vi "Select INSTR Dialog.vi"() -> (0 "Cancel":bool, 1 "element":string)   [LabVIEW 2010]
doc: "This VI scans for connected USB test and measurement devices. All found devices are shown in a list, where the user can select one of the connected devices. \nOK initialice selected device\nRESCAN look again for connected devices \nCANCEL abort application"
panel:
  in  "Rescan":bool
  in  "Cancel Button":bool
  in  "OK":bool
  in  "Select":i32(listbox) caption="Select Device from List and Press OK"
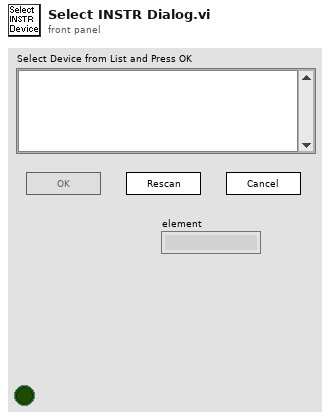
[diagram p1: front panel]
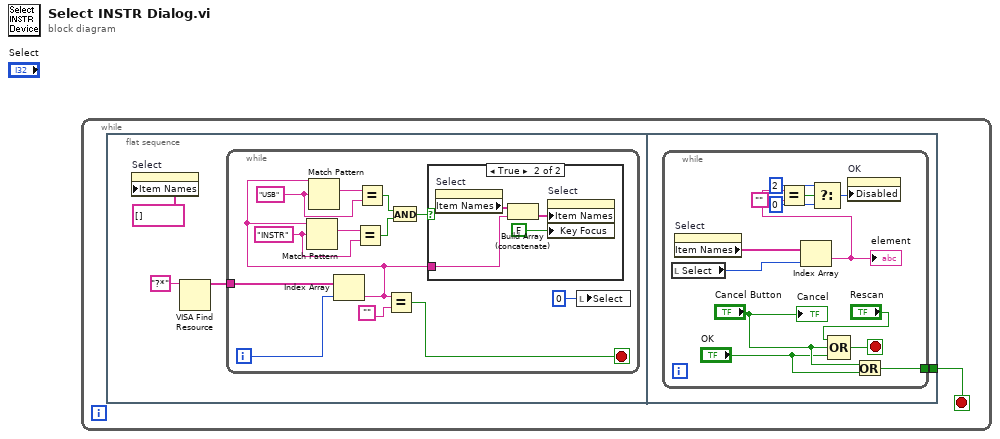
[diagram p0: block diagram]
diagram:
  n1 = while {
    stop <- w1 stop-if-true
    n2 = flat-sequence {
      tunnel: [w22] -> w1
      frame #0 {
        n3 = property on="Select" class="LstBox (strict)"("Item Names"=string[] [] ("Empty")) -> ()  [unwired: 2 in, 2 out]
        n4 = VISA Find Resource(11:"?*" ("expression (\"?*\")")) -> (3:w3:string[])  [unwired: 1 in, 3 out]
        n5 = while {
          tunnel: w3 -> [w9]
          i -> [w7]
          stop <- w6 stop-if-true
          w14 = "INSTR" ("regular expression")
          w12 = "USB" ("regular expression")
          n6 = Index Array(array=w9, index=w7) -> (element=w8:string)
          n7 = Match Pattern(string=w8, regular expression=w14) -> (match substring=w13:string)  [unwired: 4 out]
          n8 = Match Pattern(string=w8, regular expression=w12) -> (match substring=w11:string)  [unwired: 4 out]
          n9 = Equal?(x=w13, y=w14) -> (x = y?=w16:bool)
          n10 = Equal?(x=w11, y=w12) -> (x = y?=w15:bool)
          n11 = Equal?(x=w8, y="") -> (x = y?=w6:bool)
          n12 = And(x=w15, y=w16) -> (x .and. y?=w10:bool)
          n13 = case shown="True" w10 {
            tunnel: w8 -> [_ w18]
            frame False {
            }
            frame True {
              n14 = property on="Select" class="LstBox (strict)"() -> ("Item Names"=w20:string[])  [unwired: 2 in, 2 out]
              n15 = Build Array (concatenate)(w20, w18) -> (w19:string[])
              n16 = property on="Select" class="LstBox (strict)"("Item Names"=w19, "Key Focus"=FALSE) -> ()  [unwired: 2 in, 2 out]
            }
          }
          n17 = local write "Select"(0 ("Select Device from List and Press ok")) -> ()
        }
      }
      frame #1 {
        n18 = while {
          tunnel: [w29] -> w22
          stop <- w35 stop-if-true
          n19 = local read "Select"() -> (w34:i32)
          n20 = property on="Select" class="LstBox (strict)"() -> ("Item Names"=w33:string[])  [unwired: 2 in, 2 out]
          n21 = Index Array(array=w33, index=w34) -> (element=w26:string)
          "element" <- w26
          n22 = Equal?(x=w26, y="") -> (x = y?=w27:bool)
          n23 = Select(t=i8 2, s=w27, f=i8 0) -> (s? t:f=w28:i8)
          n24 = Compound Arithmetic op=OR("Rescan", "Cancel Button", "OK") -> (w35:bool)
          n25 = property on="OK" class="Bool"("Disabled"=w28) -> ()  [unwired: 2 in, 2 out]
          n26 = Or(x="Cancel Button", y="OK") -> (x .or. y?=w29:bool)
          "Cancel" <- "Cancel Button"
        }
      }
    }
  }
